vi "High G save to csv.vi"(11 "error in (no error)":errorcluster) -> (15 "error out":errorcluster)   [LabVIEW 2011]
uses:
  Stroker/High G/high G data GFV Action.ctl
  emi Lib/Basic/0 - General/Time/emi_Get DateTime In Seconds err & offs.vi
  emi Lib/Basic/0 - General/Time/Private/emi_Time offset holder.vi
  <vilib>/Utility/libraryn.llb/Check if File or Folder Exists.vi
  Application Structure/Options/Action GFV Settings.ctl
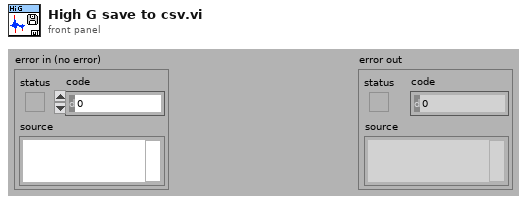
[diagram p1: front panel]
types:
  T1 = enum16{"open", "replace", "create", "open or create", "replace or create", "replace or create with confirmation"}
  T2 = enum16{"Date & Time w ms", "Date & Time", "Time w ms", "Time", "Date", "Non"}
  T3 = typedef "high G data GFV Action.ctl" = enum16{"Init", "Add data", "Get"}
  T4 = typedef "Action GFV Settings.ctl" = enum16{"Init", "Get From INI", "Put In INI", "Get Settings", "Get Update Index", "Set Setting"}
  T5 = typedef "Options  All pages and custom.ctl" = cluster{"P 1 (App)":T6, "P 2":T7, "P 3":T8, "P 4":T10, "P 5":T13, "P 6 (Err)":T14, "P 7 (Expert)":T15, "C 1":T17, "C 2":T18}
  T6 = typedef "Options Page 1 (App).ctl" = cluster{"Result files":path, "PCP Interface":string, "Modem Interface":string}
  T7 = typedef "Options Page 2.ctl" = cluster{"Audible Alarm":bool, "Force alarm on Technical":bool, "Force alarm on HH":bool, "Force alarm on LL":bool, "Force alarm on H":bool, "Force alarm on L":bool}
  T8 = typedef "Options Page 3.ctl" = cluster{"Min resistance":dbl, "Max resistance":dbl, "PCP/PSU range":T9, "Max voltage jump":dbl, "Maximum resistance change":dbl}
  T9 = typedef "PCP type List.ctl" = enum16{"0 - 350V", "0 - 450V", "0 - 600V"}
  T10 = typedef "Options Page 4.ctl" = cluster{"relay 1":dbl, "Relay 2":dbl, "Solenoid limit":dbl, "Force det.":T11, "Stroke force lim.":dbl, "Pressure SLIPS":dbl, "Tacometer puls":dbl, "Stroke force":T12}
  T11 = typedef "Stroke force selector.ctl" = enum16{"Stroke in = node 1", "Strok out = node 1"}
  T12 = typedef "Stroke force calculation.ctl" = enum16{"Node 1 minus Node 2", "Node 2 minus Node 1"}
  T13 = typedef "Options Page 5.ctl" = cluster{"Placeholder":bool}
  T14 = typedef "Options Page 6 (Err).ctl" = cluster{"Error and event files":path}
  T15 = typedef "Options Page 7 (Expert).ctl" = cluster{"Show Debug":bool, "Log debug messages":bool, "Aditional debug messages":bool, "enumCANCOM":bool, "AutoLogOn":bool, "Buffer size":i32, "Modem sim":T16, "Modem baud":u16, "Upd regular data":bool}
  T16 = typedef "Modem simulation setup.ctl" = cluster{"Modem dealay sim":bool, "Sim baud Tx":u16, "Bit Error fraction Tx":dbl, "Sim baud Rx":u16, "Bit Error fraction Rx":dbl}
  T17 = typedef "Options Custom 1.ctl" = cluster{"Placeholder":bool}
  T18 = typedef "Options Custom 2.ctl" = cluster{"Placeholder":bool}
  T19 = typedef "Project infor with project path.ctl" = cluster{"Project path":path, "data":T20, "Comment":string}
  T20 = typedef "Project in icluster.ctl" = cluster{"Job and Site":T21, "Tool":T23}
  T21 = typedef "Job and site cluster.ctl" = cluster{"Project Name":string, "Client Company":string, "Field":string, "Rig":string, "Country":T22}
  T22 = typedef "List of all contrys(combo box).ctl" = string
  T23 = typedef "Tool registration ID.ctl" = cluster{"Tractor type":string, "Tool":string, "Serial #":string}
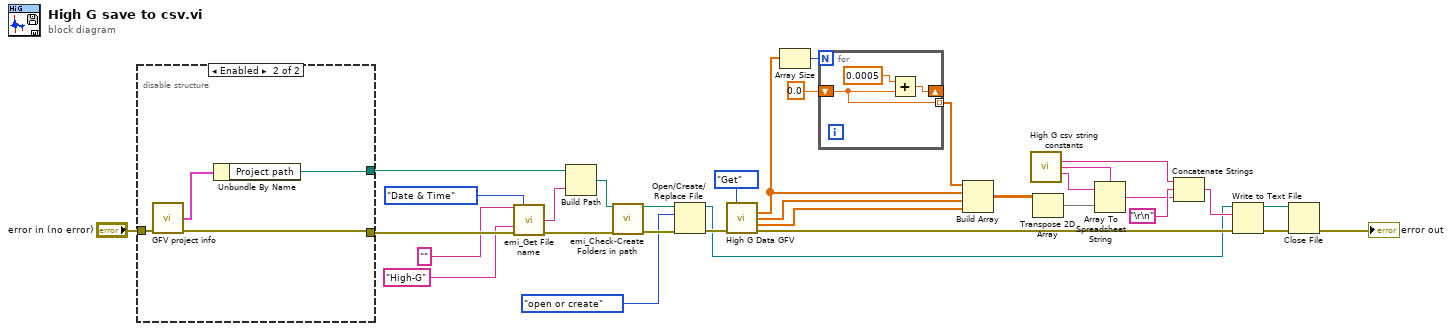
[diagram p0: block diagram]
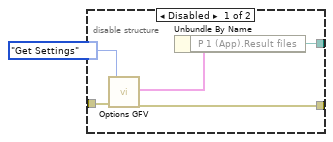
[diagram p2: hidden frame]
diagram:
  n1 = disable-structure shown="Enabled" {
    disable-tunnel: "error in (no error)" -> [w38 w42]
    disable-tunnel: [w35 w41] -> w31
    disable-tunnel: [w34 w39] -> w30
    frame Disabled {
      n2 = call "Options GFV.vi"("error in (no error)"=w38, "Action(Get Settings)"=Action_GFV_Settings."Get Settings") -> ("Options"=w36:T5, "error out"=w35:errorcluster)  [unwired: 15 in, 1 out]
      n3 = Unbundle By Name(w36) -> ("P 1 (App).Result files"=w34:path)
    }
    frame Enabled {
      n4 = call "GFV project info.vi"("error in (no error)"=w42) -> ("Project info out"=w40:T19, "error out"=w41:errorcluster)  [unwired: 13 in]
      n5 = Unbundle By Name(w40) -> ("Project path"=w39:path)
    }
  }
  n6 = call "emi_Get File name.vi"("pre date string(\"\")"="" ("pre date string(\"\")"), "Time format(Data & Time)"=T2."Date & Time", "type name(\"dat\")"="High-G" ("type name(\"dat\")"), "error in (no error)"=w31) -> ("concatenated string"=w29:string, "error out"=w25:errorcluster)  [unwired: 10 in]
  n7 = Build Path(base path=w30, name or relative path=w29) -> (appended path=w24:path)
  n8 = call "emi_Check-Create Folders in path.vi"("Path including file"=w24, "error in (no error)"=w25) -> ("Path out"=w22:path, "error out"=w23:errorcluster)  [unwired: 11 in, 1 out]
  n9 = Open/Create/Replace File(file path (use dialog)=w22, error in=w23, operation (0:open)=T1."open or create") -> (refnum out=w4:refnum<file>, error out=w20:errorcluster)  [unwired: 3 in, 1 out]
  n10 = call "High G Data GFV.vi"("Action"=high_G_data_GFV_Action."Get", "error in (no error)"=w20) -> ("X axis"=w9:dbl[], "Y axis"=w8:dbl[], "Z axis"=w7:dbl[], "error out"=w6:errorcluster)  [unwired: 9 in, 1 out]
  n11 = Array Size(array=w9) -> (size(s)=w12:i32)
  n12 = for {
    N: w12 -> [_]
    tunnel: [w45] -> w10 mode=indexing
    shift-right: [w44] -> _
    shift-left: 0.0 -> [w45]
    n13 = Add(x=0.0005, y=w45) -> (x+y=w44:dbl)
  }
  n14 = Build Array(w10, w9, w8, w7) -> (w13:dbl[][])
  n15 = call "High G csv string constants.vi"() -> ("Header"=w18:string, "Delimiter"=w19:string, "Format string"=w14:string)  [unwired: 12 in, 1 out]
  n16 = Transpose 2D Array(2D array=w13) -> (transposed array=w16:dbl[][])
  n17 = Array To Spreadsheet String(delimiter (Tab)=w19, array=w16, 3:w14) -> (spreadsheet string=w15:string)
  n18 = Concatenate Strings(w18, "\r\n", w15) -> (w5:string)
  n19 = Write to Text File(file (use dialog)=w4, text=w5, error in=w6) -> (refnum out=w2:refnum<file>, error out=w3:errorcluster)  [unwired: 1 in, 1 out]
  n20 = Close File(refnum=w2, error in=w3) -> (error out=→"error out":errorcluster)  [unwired: 1 out]
